vi "From Variant.vi"(8 "error in (no error)":errorcluster, 10 "Variant":variant, 11 "Abs_Boolean in":refnum<class "Abs_Boolean.lvclass">) -> (0 "error out":errorcluster, 3 "Abs_Boolean out":refnum<class "Abs_Boolean.lvclass">)   [LabVIEW 2021, in "Abs_Boolean.lvclass"]
uses:
  Abs_Boolean.lvclass
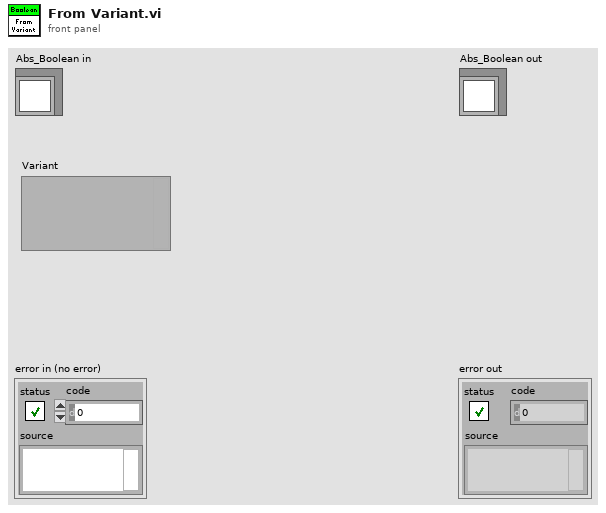
[diagram p1: front panel]
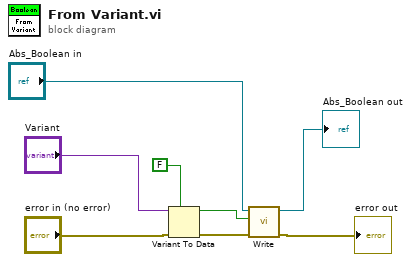
[diagram p0: block diagram]
diagram:
  n1 = Variant To Data(error in="error in (no error)", type=FALSE, Variant="Variant") -> (data=w1:bool, error out=w7:errorcluster)
  n2 = call-dynamic "Write.vi"("error in (no error)"=w7, "Boolean"=w1, "Boolean in"="Abs_Boolean in") -> ("error out"=→"error out":errorcluster, "Boolean out"=→"Abs_Boolean out":refnum<class "Abs_Boolean.lvclass">)  [unwired: 7 in]
